vi "RisingFlankCount.vi"(8 "2nd sample":bool, 9 "1st sample":bool) -> (3 "Flank count":u16)   [LabVIEW 2012]
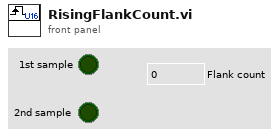
[diagram p1: front panel]
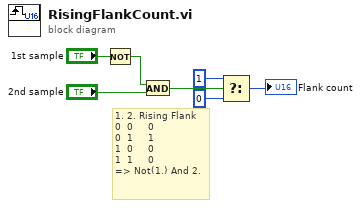
[diagram p0: block diagram]
diagram:
  # "1. 2. Rising Flank\n0  0     0\n0  1     1\n1  0     0\n1  1     0\n=> Not(1.) And 2."
  n1 = Not(x="1st sample") -> (.not. x?=w5:bool)
  n2 = And(x=w5, y="2nd sample") -> (x .and. y?=w4:bool)
  n3 = Select(t=u16 1, s=w4, f=u16 0) -> (s? t:f=→"Flank count":u16)
